vi "getServerNot.vi"(8 "error in (no error)":errorcluster, 11 "TcpServer in":refnum<class "TcpServer.lvclass">) -> (0 "error out":errorcluster, 3 "TcpServer out":refnum<class "TcpServer.lvclass">)   [LabVIEW 2018, in "TcpServer.lvclass"]
doc: "Get the notification from TCP Server that TCP Client connects or disconnects and then send an user event to the Component."
uses:
  TcpServer.lvclass
  TcpServer.lvclass/TcpServer.ctl
  TcpServerBase/TcpServerBase.lvclass/TcpServerBase.ctl
  TcpServerCmd/TcpServerCmd.lvclass
  home/pcortes/github/ts_labview_tcp_json/src/TcpServerBase/TcpServerBase.lvclass
  TcpServerTel/TcpServerTel.lvclass
  TcpServerBase/TcpServerBase.lvclass
panel:
  out "send user event":bool
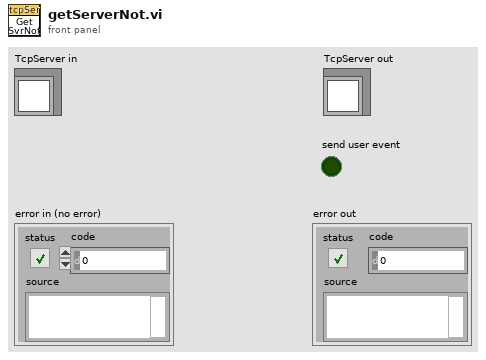
[diagram p1: front panel]
types:
  T1 = cluster{"connectionStatus":bool, "errorSource":string}
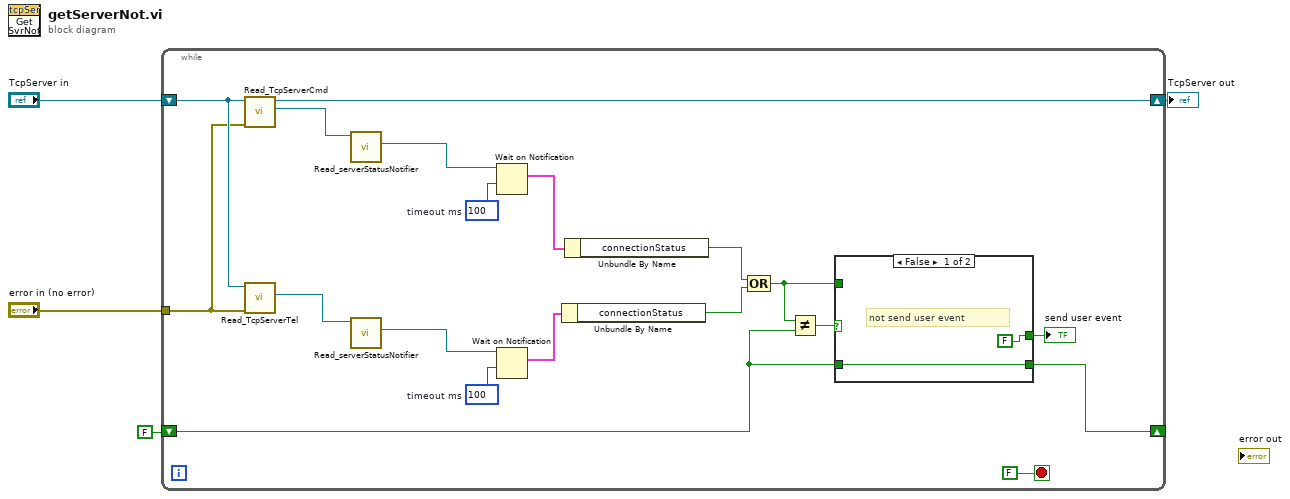
[diagram p0: block diagram]
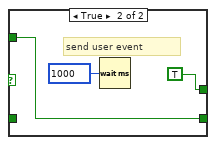
[diagram p2: hidden frame]
diagram:
  n1 = while {
    tunnel: "error in (no error)" -> [w21]
    shift-right: [w22] -> w3
    shift-left: "TcpServer in" -> [w23]
    shift-right: [w7] -> _
    shift-left: FALSE -> [w5]
    stop <- FALSE stop-if-true
    w14 = 100  # timeout ms
    w18 = 100  # timeout ms
    n2 = call "Read_TcpServerCmd.vi"("error in (no error)"=w21, "TcpServer in"=w23) -> ("TcpServerCmd.lvclass"=w20:refnum<class "TcpServerCmd.lvclass">, "TcpServer out"=w22:refnum<class "TcpServer.lvclass">)  [unwired: 7 in, 1 out]
    n3 = call "Read_TcpServerTel.vi"("error in (no error)"=w21, "TcpServer in"=w23) -> ("TcpServerTel.lvclass"=w19:refnum<class "TcpServerTel.lvclass">)  [unwired: 7 in, 2 out]
    n4 = call "Read_serverStatusNotifier.vi"("TcpServerBase in"=w20) -> ("serverStatusNotifier"=w16:refnum<notifier>)  [unwired: 8 in, 2 out]
    n5 = call "Read_serverStatusNotifier.vi"("TcpServerBase in"=w19) -> ("serverStatusNotifier"=w13:refnum<notifier>)  [unwired: 8 in, 2 out]
    n6 = Wait on Notification(notifier=w16, timeout in ms (-1)=w18) -> (notification=w17:T1)  [unwired: 2 in, 3 out]
    n7 = Wait on Notification(notifier=w13, timeout in ms (-1)=w14) -> (notification=w15:T1)  [unwired: 2 in, 3 out]
    n8 = Unbundle By Name(w15) -> ("connectionStatus"=w11:bool)
    n9 = Unbundle By Name(w17) -> ("connectionStatus"=w12:bool)
    n10 = Compound Arithmetic op=OR(w12, w11) -> (w6:bool)
    n11 = Not Equal?(x=w6, y=w5) -> (x != y?=w8:bool)
    n12 = case shown="False" w8 {
      tunnel: [FALSE TRUE] -> w9
      tunnel: [w24 w26] -> w7
      tunnel: w6 -> [_ w26]
      tunnel: w5 -> [w24 _]
      frame False {
        # "not send user event"
      }
      frame True {
        # "send user event"
        n13 = Wait (ms)(milliseconds to wait=u32 1000) -> ()  [unwired: 1 out]
      }
    }
    "send user event" <- w9
  }
  "TcpServer out" <- w3
